vi "macro_Rotation3d_RollPitchYaw_Rad.vi"   [LabVIEW 2019, in "Trajectory_Library.lvlib"]
uses:
  Trajectory_Library.lvlib
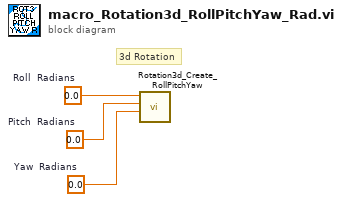
[diagram p0: block diagram]
diagram:
  w1 = 0.0  # Roll  Radians
  w2 = 0.0  # Pitch  Radians
  w3 = 0.0  # Yaw  Radians
  # "3d Rotation"
  n1 = call "Rotation3d_Create_RollPitchYaw.vi"("Yaw"=w3, "Pitch"=w2, "Roll"=w1) -> ()  [unwired: 8 in, 1 out]
